vi "Obtain Request Events.vi"(8 "error in":errorcluster, 10 "Create New? (F)":bool) -> (0 "error out":errorcluster, 2 "Stepper Request Events":T1)   [LabVIEW 2025, in "Stepper.lvlib"]
doc: "This VI Obtains/Creates the Requests events that will be used for other modules to communicate with the module that owns this VI. These Requests events will be accessed only via Public API methods for this module.\n\n<b>NOTE</b>: The contents of this VI are automatically generated and modified by the <b>Tools > DQMH Consortium > DQMH</b> utilities. Consider using those utilities instead of making your own modifications to this VI.\n_____\nBased on DQMH Dev Tools: Project Template 7.1.2.1547."
uses:
  Stepper.lvlib
  Request Events--cluster.ctl
  Stop Argument--cluster.ctl
  Show Panel Argument--cluster.ctl
  Hide Panel Argument--cluster.ctl
  Show Diagram Argument--cluster.ctl
  Get Module Execution Status Argument--cluster.ctl
  close Argument--cluster.ctl
  close (Reply Payload)--cluster.ctl
  init Argument--cluster.ctl
  init (Reply Payload)--cluster.ctl
  init driver Argument--cluster.ctl
  init driver (Reply Payload)--cluster.ctl
  Clear Motor Error Argument--cluster.ctl
  Clear Motor Error (Reply Payload)--cluster.ctl
  read config Argument--cluster.ctl
  read config (Reply Payload)--cluster.ctl
  Read Angle Argument--cluster.ctl
  Read Angle (Reply Payload)--cluster.ctl
  Jog Argument--cluster.ctl
  Jog (Reply Payload)--cluster.ctl
  Go To Angle Argument--cluster.ctl
  Go To Angle (Reply Payload)--cluster.ctl
panel:
  # "NOTE: The contents of this VI are automatically generated and modified by the Tools > DQMH Consortium > DQMH utilities. Consider using those utilities instead of making your own modifications to this VI."
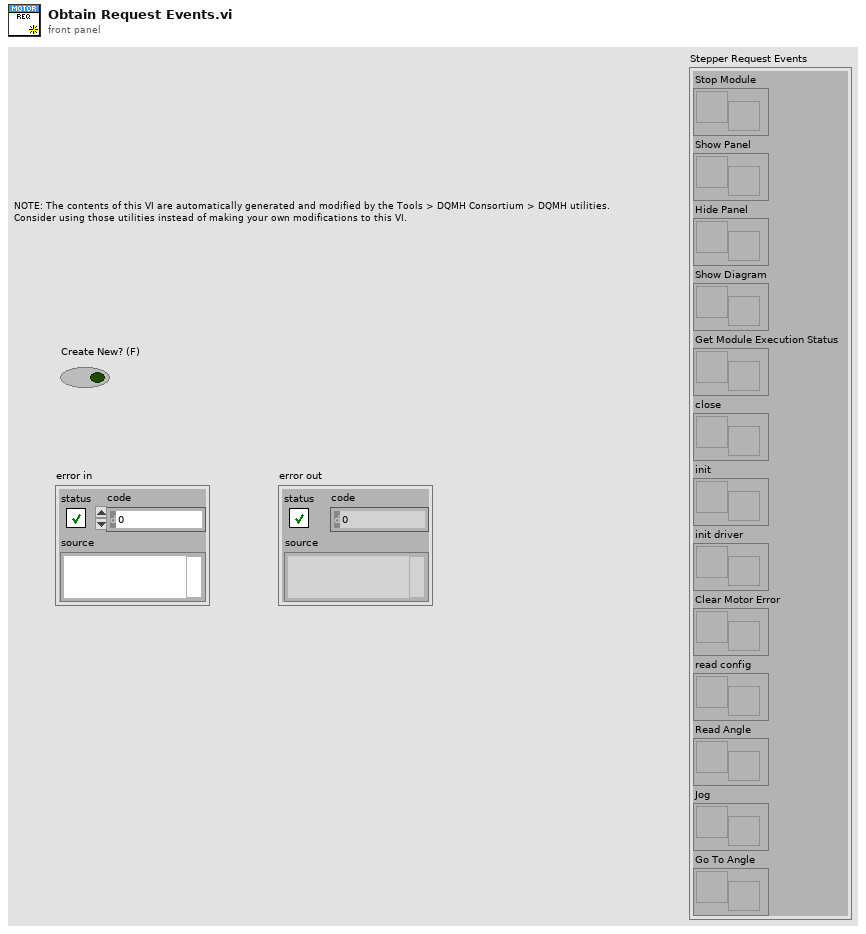
[diagram p1: front panel]
types:
  T1 = typedef "Stepper.lvlib/Request Events--cluster.ctl" = cluster{"Stop Module":refnum<user-event>, "Show Panel":refnum<user-event>, "Hide Panel":refnum<user-event>, "Show Diagram":refnum<user-event>, "Get Module Execution Status":refnum<user-event>, "close":refnum<user-event>, "init":refnum<user-event>, "init driver":refnum<user-event>, "Clear Motor Error":refnum<user-event>, "read config":refnum<user-event>, "Read Angle":refnum<user-event>, "Jog":refnum<user-event>, "Go To Angle":refnum<user-event>}
  T2 = typedef "Stepper.lvlib/Go To Angle Argument--cluster.ctl" = cluster{"Module ID":i32, "Angle":dbl, "Velocity [rpm]":i32, "Pause Time [ms]":i32, "Wait Notifier":refnum<notifier>, "wait for reply":bool}
  T3 = typedef "Stepper.lvlib/Jog Argument--cluster.ctl" = cluster{"Module ID":i32, "CCW? (T)":bool, "[rpm]":u16, "Wait Notifier":refnum<notifier>, "wait for reply":bool}
  T4 = typedef "Stepper.lvlib/Read Angle Argument--cluster.ctl" = cluster{"Module ID":i32, "Wait Notifier":refnum<notifier>, "wait for reply":bool}
  T5 = typedef "Stepper.lvlib/read config Argument--cluster.ctl" = cluster{"Module ID":i32, "config file path":path, "Wait Notifier":refnum<notifier>, "wait for reply":bool}
  T6 = typedef "Stepper.lvlib/Clear Motor Error Argument--cluster.ctl" = cluster{"Module ID":i32, "Wait Notifier":refnum<notifier>, "wait for reply":bool}
  T7 = typedef "Stepper.lvlib/init driver Argument--cluster.ctl" = cluster{"Module ID":i32, "Wait Notifier":refnum<notifier>, "wait for reply":bool}
  T8 = typedef "Stepper.lvlib/init Argument--cluster.ctl" = cluster{"Module ID":i32, "Wait Notifier":refnum<notifier>, "wait for reply":bool}
  T9 = typedef "Stepper.lvlib/close Argument--cluster.ctl" = cluster{"Module ID":i32, "Wait Notifier":refnum<notifier>, "wait for reply":bool}
  T10 = typedef "Stepper.lvlib/Get Module Execution Status Argument--cluster.ctl" = cluster{"Module ID":i32, "Running?":bool}
  T11 = typedef "Stepper.lvlib/Show Diagram Argument--cluster.ctl" = cluster{"Module ID":i32, "Debug?":bool}
  T12 = typedef "Stepper.lvlib/Show Panel Argument--cluster.ctl" = cluster{"Module ID":i32, "Show Panel?":bool}
  T13 = typedef "Stepper.lvlib/Hide Panel Argument--cluster.ctl" = cluster{"Module ID":i32, "Hide Panel?":bool}
  T14 = typedef "Stepper.lvlib/Stop Argument--cluster.ctl" = cluster{"Module ID":i32, "Origin":string, "Exit via Stop Module Req?":bool, "Wait for Module to stop?":bool}
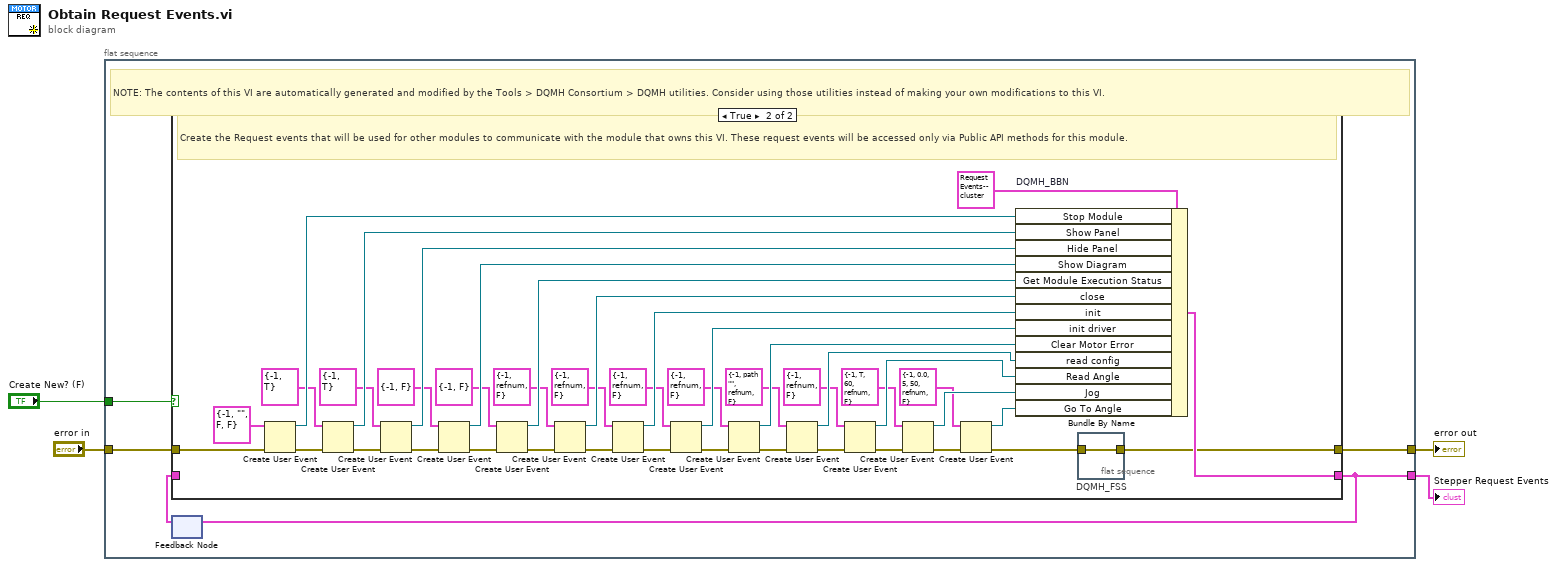
[diagram p0: block diagram]
diagram:
  n1 = flat-sequence {
    tunnel: [w9] -> w4
    tunnel: "error in" -> [w8]
    tunnel: [w6] -> w2
    tunnel: "Create New? (F)" -> [w5]
    frame #0 {
      # "NOTE: The contents of this VI are automatically generated and modified by the Tools > DQMH Consortium > DQMH utilities. Consider using those utilities instead of making your own modifications to this VI."
      n2 = feedback #1() -> (w7:T1)  [unwired: 1 in]
      n3 = case shown="True" w5 {
        tunnel: [w10 w42] -> w9
        tunnel: w8 -> [w10 w54]
        tunnel: [w11 w51] -> w6
        tunnel: w7 -> [w11 _]
        frame False {
        }
        frame True {
          # "Create the Request events that will be used for other modules to communicate with the module that owns this VI. These request events will be accessed only via Public API methods for this module."
          n4 = Create User Event(user event datatype=T14 {"Module ID"=-1, "Origin"="", "Exit via Stop Module Req?"=FALSE, "Wait for Module to stop?"=FALSE} ("Stop Argument"), error in=w54) -> (user event=w52:refnum<user-event>, error out=w49:errorcluster)
          n5 = Create User Event(user event datatype=T12 {"Module ID"=-1, "Show Panel?"=TRUE} ("Show Panel Argument"), error in=w49) -> (user event=w48:refnum<user-event>, error out=w46:errorcluster)
          n6 = Create User Event(user event datatype=T13 {"Module ID"=-1, "Hide Panel?"=TRUE} ("Hide Panel"), error in=w46) -> (user event=w45:refnum<user-event>, error out=w44:errorcluster)
          n7 = Create User Event(user event datatype=T11 {"Module ID"=-1, "Debug?"=FALSE} ("Show Diagram Argument"), error in=w44) -> (user event=w40:refnum<user-event>, error out=w41:errorcluster)
          n8 = Create User Event(user event datatype=T10 {"Module ID"=-1, "Running?"=FALSE} ("Get Module Execution Status Argument"), error in=w41) -> (user event=w37:refnum<user-event>, error out=w38:errorcluster)
          n9 = Create User Event(user event datatype=T9 {"Module ID"=-1, "Wait Notifier"=refnum, "wait for reply"=FALSE} ("close Argument"), error in=w38) -> (user event=w34:refnum<user-event>, error out=w35:errorcluster)
          n10 = Create User Event(user event datatype=T8 {"Module ID"=-1, "Wait Notifier"=refnum, "wait for reply"=FALSE} ("init Argument"), error in=w35) -> (user event=w31:refnum<user-event>, error out=w32:errorcluster)
          n11 = Create User Event(user event datatype=T7 {"Module ID"=-1, "Wait Notifier"=refnum, "wait for reply"=FALSE} ("init driver Argument"), error in=w32) -> (user event=w28:refnum<user-event>, error out=w29:errorcluster)
          n12 = Create User Event(user event datatype=T6 {"Module ID"=-1, "Wait Notifier"=refnum, "wait for reply"=FALSE} ("Clear Motor Error Argument"), error in=w29) -> (user event=w25:refnum<user-event>, error out=w26:errorcluster)
          n13 = Create User Event(user event datatype=T5 {"Module ID"=-1, "config file path"=path "", "Wait Notifier"=refnum, "wait for reply"=FALSE} ("read config Argument"), error in=w26) -> (user event=w22:refnum<user-event>, error out=w23:errorcluster)
          n14 = Create User Event(user event datatype=T4 {"Module ID"=-1, "Wait Notifier"=refnum, "wait for reply"=FALSE} ("Read Angle Argument"), error in=w23) -> (user event=w19:refnum<user-event>, error out=w20:errorcluster)
          n15 = Create User Event(user event datatype=T3 {"Module ID"=-1, "CCW? (T)"=TRUE, "[rpm]"=60, "Wait Notifier"=refnum, "wait for reply"=FALSE} ("Jog Argument"), error in=w20) -> (user event=w16:refnum<user-event>, error out=w17:errorcluster)
          n16 = Create User Event(user event datatype=T2 {"Module ID"=-1, "Angle"=0.0, "Velocity [rpm]"=5, "Pause Time [ms]"=50, "Wait Notifier"=refnum, "wait for reply"=FALSE} ("Go To Angle Argument"), error in=w17) -> (user event=w13:refnum<user-event>, error out=w14:errorcluster)
          n17 = Bundle By Name "DQMH_BBN"(cluster=T1 {"Stop Module"=refnum, "Show Panel"=refnum, "Hide Panel"=refnum, "Show Diagram"=refnum, "Get Module Execution Status"=refnum, "close"=refnum, "init"=refnum, "init driver"=refnum, "Clear Motor Error"=refnum, "read config"=refnum, "Read Angle"=refnum, "Jog"=refnum, "Go To Angle"=refnum} ("output cluster"), "Stop Module"=w52, "Show Panel"=w48, "Hide Panel"=w45, "Show Diagram"=w40, "Get Module Execution Status"=w37, "close"=w34, "init"=w31, "init driver"=w28, "Clear Motor Error"=w25, "read config"=w22, "Read Angle"=w19, "Jog"=w16, "Go To Angle"=w13) -> (w51:T1)
          n18 = flat-sequence "DQMH_FSS" {
            tunnel: w14 -> [w55]
            tunnel: [w55] -> w42
            frame #0 {
            }
          }
        }
      }
      n19 = feedback-in #1(w6) -> ()
    }
  }
  "Stepper Request Events" <- w2
  "error out" <- w4
